vi "Begin.vi"(8 "error in":errorcluster) -> (0 "error out":errorcluster)   [LabVIEW 2018]
doc: "Called before other user functions, this VI is expected to open initial I/O refnums, load in file data, and do all program initialization. Notice that the <B>error out</B> terminal is simply used for data flow. Wiring it to other structures or subVIs ensures that this VI runs first."
uses:
  <vilib>/Rock Robotics/WPI/DriverStation/WPI_DriverStationRobotMode2.ctl
  Classes/Configuration File/Configuration File.lvclass
  TypeDefs/RobotObjects.ctl
  Classes/Drive/Drive.lvclass
  Classes/Pnematics control/Pneumatics.lvclass
  Classes/Vision/Vision.lvclass
  Classes/Joysticks/Joysticks.lvclass
  Classes/Elevator/Elevator.lvclass
  Classes/Hatch/Hatch.lvclass
  Classes/Cargo/Cargo.lvclass
  Classes/Joysticks/Joysticks.lvclass/Joysticks.ctl
  Classes/Joysticks/Public Methods/Write Sensitivity(x).vi
  Classes/Joysticks/Public Methods/Write Sensitivity(y).vi
  Robot Global Data.vi
  RobotGlobal.vi
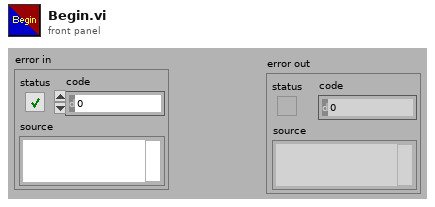
[diagram p1: front panel]
types:
  T1 = typedef "WPI_DriverStationRobotMode2.ctl" = enum16{"Autonomous Disabled", "Autonomous Enabled", "Teleop Disabled", "Teleop Enabled", "Disconnected", "Finish", "Test Disabled", "Test Enabled", "Emergency Stopped"}
  T2 = typedef "RobotObjects.ctl" = cluster{"Drive.lvclass":refnum<class "Drive.lvclass">, "Pneumatics.lvclass":refnum<class "Pneumatics.lvclass">, "Vision.lvclass":refnum<class "Vision.lvclass">, "Joysticks.lvclass":refnum<class "Joysticks.lvclass">, "Elevator.lvclass":refnum<class "Elevator.lvclass">, "Hatch.lvclass":refnum<class "Hatch.lvclass">, "Cargo.lvclass":refnum<class "Cargo.lvclass">}
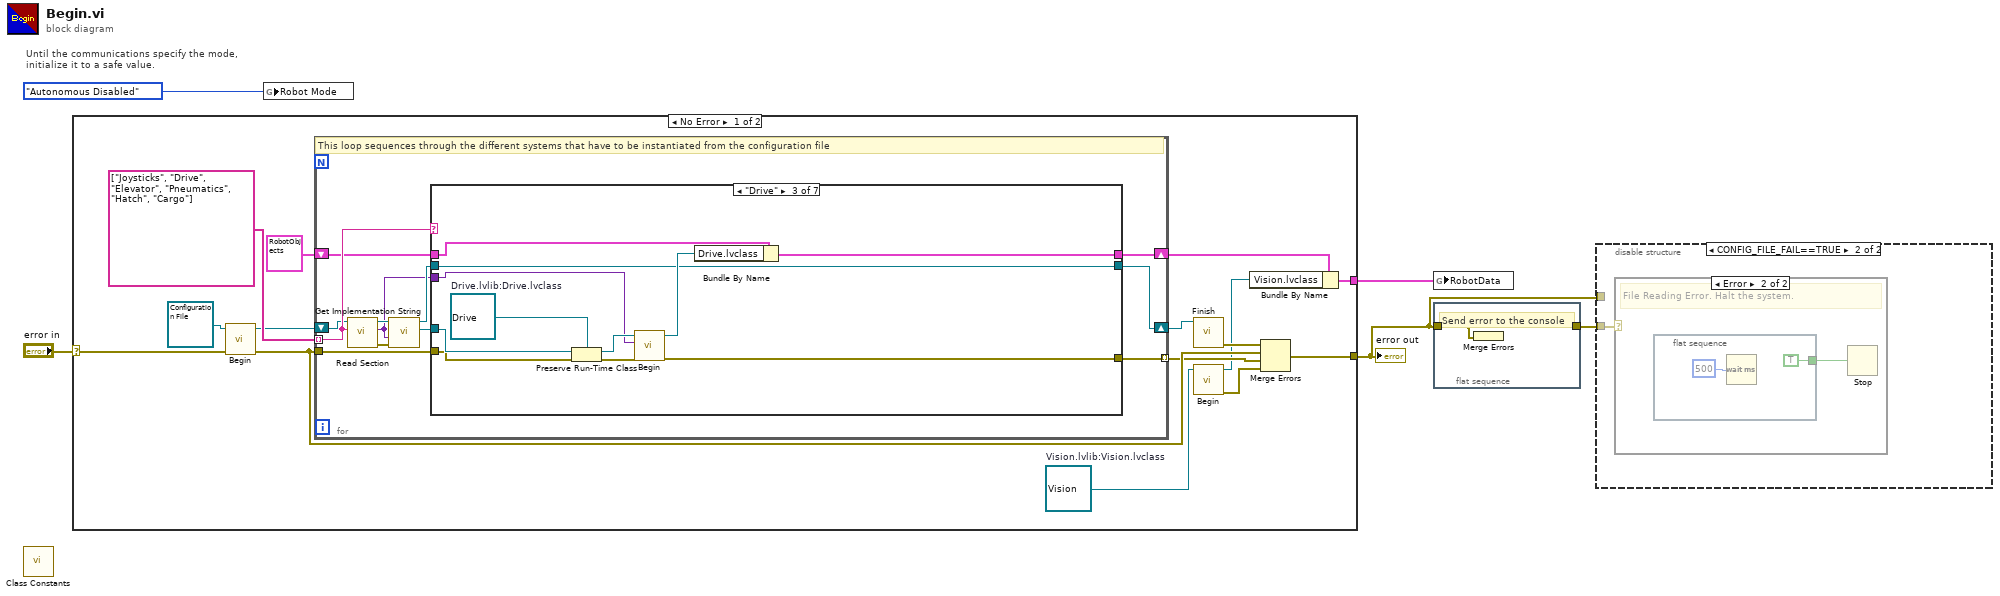
[diagram p0: block diagram]
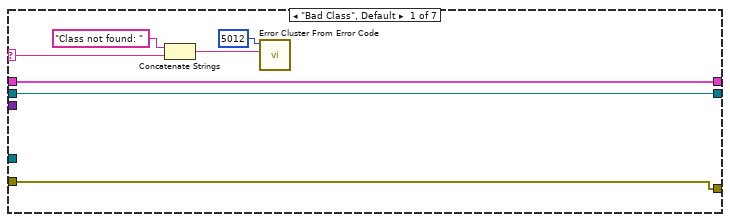
[diagram p4: hidden frame]
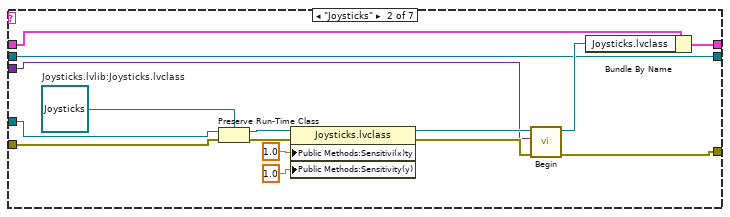
[diagram p5: hidden frame]
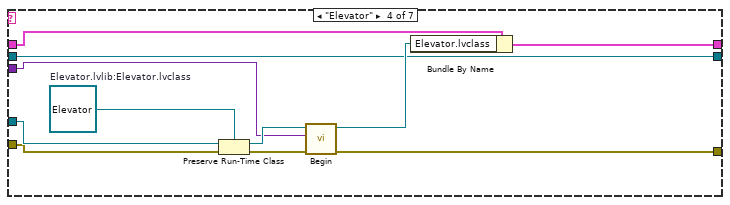
[diagram p6: hidden frame]
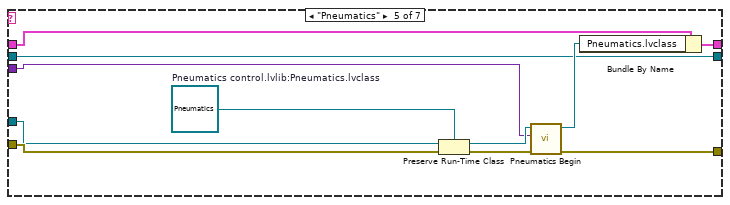
[diagram p7: hidden frame]
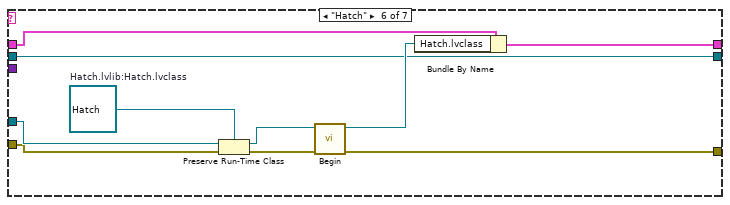
[diagram p8: hidden frame]
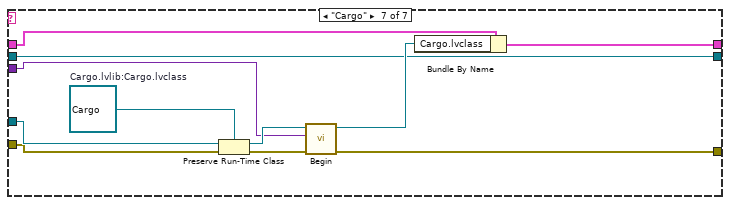
[diagram p9: hidden frame]
diagram:
  # "Until the communications specify the mode,\ninitialize it to a safe value."
  n1 = call "Class Constants.vi"() -> ()  [unwired: 12 in]
  n2 = case shown="No Error" "error in" {
    selector: "error in" -> [w17 w109]
    tunnel: [w9 _] -> w1
    tunnel: [w18 w109] -> w3
    frame No Error {
      w8 = refnum<class "Vision.lvclass"> refnum  # Vision.lvlib:Vision.lvclass
      n3 = call-dynamic "Begin.vi"("error in (no error)"=w17, "Configuration File in"=refnum<class "Configuration File.lvclass"> refnum) -> ("error out"=w13:errorcluster, "Configuration File out"=w12:refnum<class "Configuration File.lvclass">)  [unwired: 8 in]
      n4 = for {
        tunnel: string[] ["Joysticks", "Drive", "Elevator", "Pneumatics", "Hatch", "Cargo"] -> [w32] mode=indexing
        tunnel: w13 -> [w26]
        shift-right: [w25] -> w15
        shift-left: T2 {"Drive.lvclass"=refnum, "Pneumatics.lvclass"=refnum, "Vision.lvclass"=refnum, "Joysticks.lvclass"=refnum, "Elevator.lvclass"=refnum, "Hatch.lvclass"=refnum, "Cargo.lvclass"=refnum} -> [w24]
        shift-right: [w22] -> w11
        shift-left: w12 -> [w23]
        tunnel: [w21] -> w10 mode=indexing
        # "This loop sequences through the different systems that have to be instantiated from the configuration file"
        n5 = call-dynamic "Read Section.vi"("Section Name"=w32, "Configuration File in"=w23) -> ("error out"=w30:errorcluster, "Data Out"=w28:variant, "Configuration File out"=w31:refnum<class "Configuration File.lvclass">)  [unwired: 6 in, 1 out]
        n6 = call-dynamic "Get Implementation String.vi"("error in (no error)"=w30, "Data In"=w28, "Configuration File in"=w31) -> ("Class Out"=w27:refnum<class>, "Configuration File out"=w29:refnum<class "Configuration File.lvclass">)  [unwired: 6 in, 1 out]
        n7 = case shown="\"Drive\"" w32 {
          selector: w32 -> [w33 _ _ _ _ _ _]
          tunnel: w29 -> [w38 w40 w55 w66 w78 w88 w98]
          tunnel: w28 -> [_ w41 w57 w67 w84 _ w100]
          tunnel: w27 -> [_ w53 w65 w76 w82 w97 w108]
          tunnel: w26 -> [w37 w52 w64 w75 w83 w96 w107]
          tunnel: [w37 w51 w62 w72 w85 w94 w104] -> w21
          tunnel: [w39 w49 w60 w70 w81 w92 w102] -> w25
          tunnel: w24 -> [w39 w50 w61 w71 w79 w93 w103]
          tunnel: [w38 w40 w55 w66 w78 w88 w98] -> w22
          frame "Bad Class", Default {
            n8 = Concatenate Strings("Class not found: " ("error message (\"\")"), w33) -> (w34:string)
            n9 = call <vilib>:"Error Cluster From Error Code.vi"("error message (\"\")"=w34, "error code (0)"=5012) -> ()  [unwired: 7 in, 1 out]
          }
          frame "Joysticks" {
            w54 = refnum<class "Joysticks.lvclass"> refnum  # Joysticks.lvlib:Joysticks.lvclass
            n10 = Preserve Run-Time Class(object in=w53, error in=w52, 2:w54) -> (object out=w45:refnum<class "Joysticks.lvclass">, error out=w43:errorcluster)
            n11 = property class="Joysticks.lvclass"(reference=w45, error in=w43, "Public Methods:Sensitivi(x)ty"=1.0 ("Sensitivi(x)ty"), "Public Methods:Sensitivity(y)"=1.0 ("Sensitivity(y)")) -> (reference out=w44:refnum<class "Joysticks.lvclass">, error out=w42:errorcluster)
            n12 = call-dynamic "Begin.vi"("error in (no error)"=w42, "Settings In"=w41, "Joysticks in"=w44) -> ("error out"=w51:errorcluster, "Joysticks out"=w48:refnum<class "Joysticks.lvclass">)  [unwired: 7 in]
            n13 = Bundle By Name(cluster=w50, "Joysticks.lvclass"=w48) -> (w49:T2)
          }
          frame "Drive" {
            w56 = refnum<class "Drive.lvclass"> refnum  # Drive.lvlib:Drive.lvclass
            n14 = Preserve Run-Time Class(object in=w65, error in=w64, 2:w56) -> (object out=w58:refnum<class "Drive.lvclass">, error out=w63:errorcluster)
            n15 = call-dynamic "Begin.vi"("error in (no error)"=w63, "Settings"=w57, "Drive in"=w58) -> ("error out"=w62:errorcluster, "Drive out"=w59:refnum<class "Drive.lvclass">)  [unwired: 7 in]
            n16 = Bundle By Name(cluster=w61, "Drive.lvclass"=w59) -> (w60:T2)
          }
          frame "Elevator" {
            w68 = refnum<class "Elevator.lvclass"> refnum  # Elevator.lvlib:Elevator.lvclass
            n17 = Preserve Run-Time Class(object in=w76, error in=w75, 2:w68) -> (object out=w74:refnum<class "Elevator.lvclass">, error out=w73:errorcluster)
            n18 = call-dynamic "Begin.vi"("error in (no error)"=w73, "Settings"=w67, "Elevator in"=w74) -> ("error out"=w72:errorcluster, "Elevator out"=w69:refnum<class "Elevator.lvclass">)  [unwired: 7 in]
            n19 = Bundle By Name(cluster=w71, "Elevator.lvclass"=w69) -> (w70:T2)
          }
          frame "Pneumatics" {
            w87 = refnum<class "Pneumatics.lvclass"> refnum  # Pneumatics control.lvlib:Pneumatics.lvclass
            n20 = Preserve Run-Time Class(object in=w82, error in=w83, 2:w87) -> (object out=w86:refnum<class "Pneumatics.lvclass">, error out=w77:errorcluster)
            n21 = call "Pneumatics Begin.vi"("error in (no error)"=w77, "Data Out"=w84, "Pneumatics in"=w86) -> ("error out"=w85:errorcluster, "Pneumatics out"=w80:refnum<class "Pneumatics.lvclass">)  [unwired: 7 in]
            n22 = Bundle By Name(cluster=w79, "Pneumatics.lvclass"=w80) -> (w81:T2)
          }
          frame "Hatch" {
            w91 = refnum<class "Hatch.lvclass"> refnum  # Hatch.lvlib:Hatch.lvclass
            n23 = Preserve Run-Time Class(object in=w97, error in=w96, 2:w91) -> (object out=w90:refnum<class "Hatch.lvclass">, error out=w95:errorcluster)
            n24 = call-dynamic "Begin.vi"("error in (no error)"=w95, "Hatch in"=w90) -> ("error out"=w94:errorcluster, "Hatch out"=w89:refnum<class "Hatch.lvclass">)  [unwired: 8 in]
            n25 = Bundle By Name(cluster=w93, "Hatch.lvclass"=w89) -> (w92:T2)
          }
          frame "Cargo" {
            w99 = refnum<class "Cargo.lvclass"> refnum  # Cargo.lvlib:Cargo.lvclass
            n26 = Preserve Run-Time Class(object in=w108, error in=w107, 2:w99) -> (object out=w106:refnum<class "Cargo.lvclass">, error out=w105:errorcluster)
            n27 = call-dynamic "Begin.vi"("error in (no error)"=w105, "Configuration In"=w100, "Cargo in"=w106) -> ("error out"=w104:errorcluster, "Cargo out"=w101:refnum<class "Cargo.lvclass">)  [unwired: 7 in]
            n28 = Bundle By Name(cluster=w103, "Cargo.lvclass"=w101) -> (w102:T2)
          }
        }
      }
      n29 = call-dynamic "Finish.vi"("Configuration File in"=w11) -> ("error out"=w19:errorcluster)  [unwired: 7 in, 3 out]
      n30 = call-dynamic "Begin.vi"("Vision in"=w8) -> ("error out"=w6:errorcluster, "Vision out"=w7:refnum<class "Vision.lvclass">)  [unwired: 9 in]
      n31 = Bundle By Name(cluster=w15, "Vision.lvclass"=w7) -> (w9:T2)
      n32 = Merge Errors(w19, w13, w10, w6) -> (w18:errorcluster)
    }
    frame Error {
    }
  }
  "error out" <- w3
  n33 = global write "Robot Global Data.vi" "Robot Mode"(WPI_DriverStationRobotMode2."Autonomous Disabled" ("Robot Mode")) -> ()
  n34 = global write "RobotGlobal.vi" "RobotData"(w1) -> ()
  n35 = flat-sequence {
    tunnel: w3 -> [w110]
    tunnel: [w110] -> w2
    frame #0 {
      # "Send error to the console"
      n36 = Merge Errors(w110) -> ()  [unwired: 1 out]
    }
  }
  n37 = disable-structure shown="CONFIG_FILE_FAIL==TRUE" {
    disable-tunnel: w3 -> [_ _]
    disable-tunnel: w2 -> [_ w111]
    frame condition #0 (active) {
      # "If the project key to halt the execution if the configuration file is wrong\nis not activated, then do nothing if we have an error at the end."
    }
    frame condition #1 {
      n38 = case shown="Error" w111 {
        frame No Error {
        }
        frame Error {
          # "File Reading Error. Halt the system."
          n39 = flat-sequence {
            tunnel: [TRUE ("stop? (T)")] -> w112
            frame #0 {
              n40 = Wait (ms)(milliseconds to wait=u32 500) -> ()  [unwired: 1 out]
            }
          }
          n41 = Stop(stop? (T)=w112) -> ()
        }
      }
    }
  }
